vi "testSumin2.vi"() -> ()   [LabVIEW 2011]
panel:
  out "Image":T1(plugin-control)
  in  "DR/R parameter":T2
  out "BlkFilePath":path
  out "stim":i32
  out "Stimuli":i32
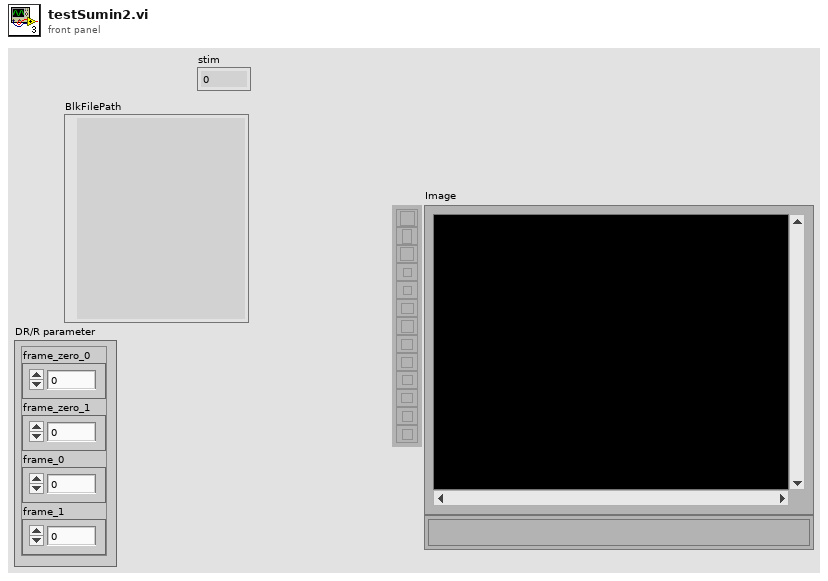
[diagram p1: front panel]
types:
  T1 = typedef "IMAQ Image.ctl" = refnum<image>
  T2 = cluster{"frame_zero_0":i32, "frame_zero_1":i32, "frame_0":i32, "frame_1":i32}
  T3 = typedef "Image Type" = u32
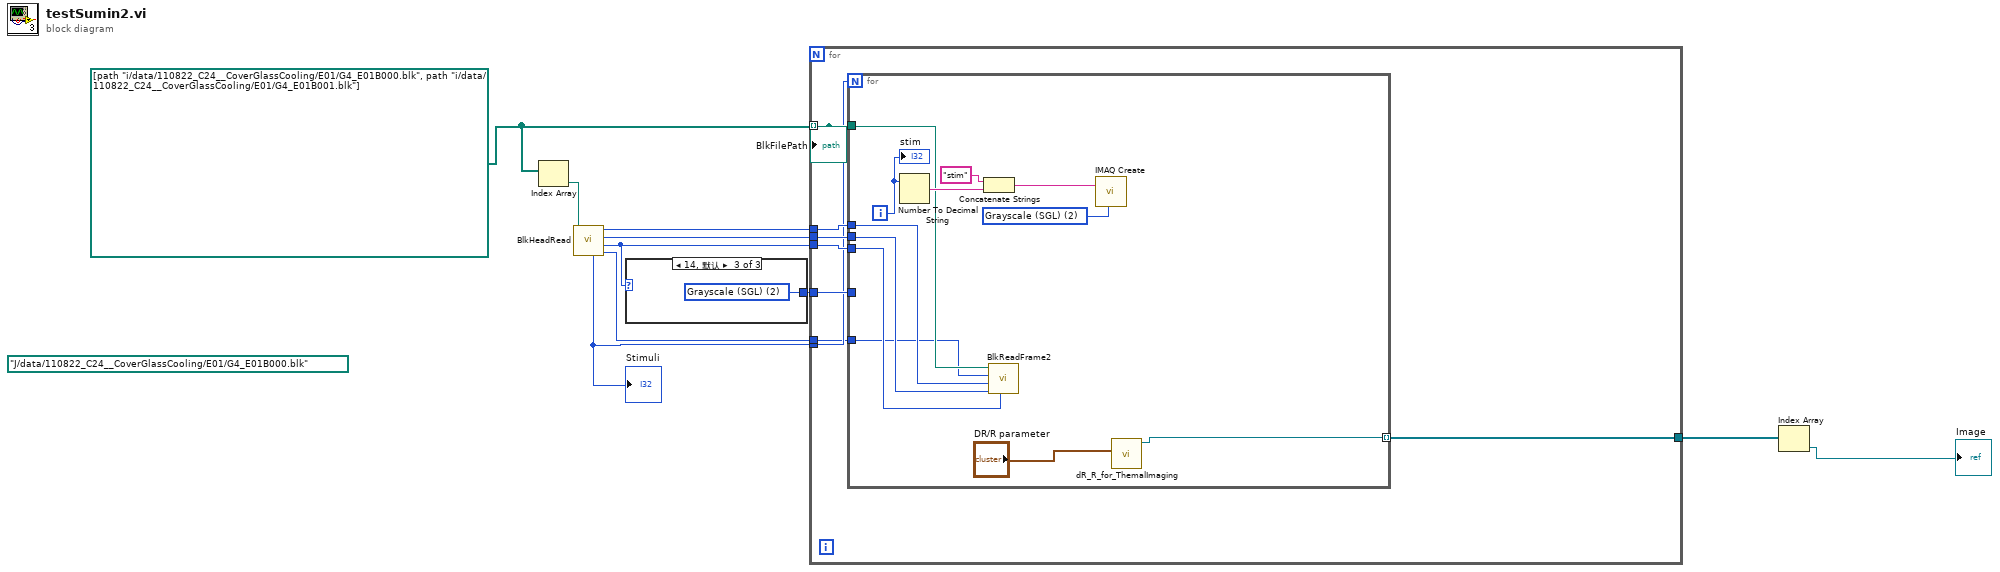
[diagram p0: block diagram]
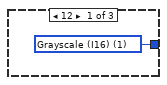
[diagram p2: hidden frame]
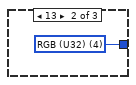
[diagram p3: hidden frame]
diagram:
  (unwired) path "J:/data/110822_C24__CoverGlassCooling/E01/G4_E01B000.blk" ("BlkFilePath")
  w4 = path[] [path "i:/data/110822_C24__CoverGlassCooling/E01/G4_E01B000.blk", path "i:/data/110822_C24__CoverGlassCooling/E01/G4_E01B001.blk"]
  n1 = Index Array(array=w4) -> (element=w3:path)  [unwired: 1 in]
  n2 = call "BlkHeadRead.vi"("BlkFilePath"=w3) -> ("FramesPerStim"=w7:i32, "datatype"=w8:i32, "FrameHeight"=w9:i32, "FrameWidth"=w10:i32, "Stimuli"=w6:i32)  [unwired: 6 in]
  "Stimuli" <- w6
  n3 = case shown="14, 默认" w8 {
    tunnel: [w11 w12 w13] -> w5
    frame 12 {
      w11 = T3 1 items=["Grayscale (U8)", "Grayscale (I16)", "Grayscale (SGL)", "Complex (CSG)", "RGB (U32)", "HSL (U32)", "RGB (U64)", "Grayscale (U16)"] ("Image Type")
    }
    frame 13 {
      w12 = T3 4 items=["Grayscale (U8)", "Grayscale (I16)", "Grayscale (SGL)", "Complex (CSG)", "RGB (U32)", "HSL (U32)", "RGB (U64)", "Grayscale (U16)"] ("Image Type")
    }
    frame 14, Default {
      w13 = T3 2 items=["Grayscale (U8)", "Grayscale (I16)", "Grayscale (SGL)", "Complex (CSG)", "RGB (U32)", "HSL (U32)", "RGB (U64)", "Grayscale (U16)"] ("Image Type")
    }
  }
  n4 = for {
    tunnel: w10 -> [w21]
    tunnel: w9 -> [w20]
    tunnel: w8 -> [w19]
    tunnel: w4 -> [w18] mode=indexing
    tunnel: w5 -> [w17]
    tunnel: w6 -> [w16]
    tunnel: w7 -> [w15]
    tunnel: [w14] -> w2
    n5 = for {
      N: w16 -> [_]
      tunnel: w18 -> [w30]
      tunnel: w21 -> [w29]
      tunnel: w20 -> [w28]
      tunnel: w19 -> [w27]
      tunnel: w17 -> [_]
      tunnel: w15 -> [w26]
      tunnel: [w22] -> w14 mode=indexing
      i -> [w33]
      w24 = T3 2 items=["Grayscale (U8)", "Grayscale (I16)", "Grayscale (SGL)", "Complex (CSG)", "RGB (U32)", "HSL (U32)", "RGB (U64)", "Grayscale (U16)"] ("Image Type")
      n6 = Number To Decimal String(number=w33) -> (decimal integer string=w32:string)  [unwired: 1 in]
      n7 = Concatenate Strings("stim" ("字符串"), w32) -> (w25:string)
      n8 = call "BlkReadFrame2.vi"("datatype"=w27, "FrameHeight"=w28, "FrameWidth"=w29, "frameNO."=w26, "BlkFilePath"=w30) -> ()  [unwired: 2 in, 3 out]
      n9 = call "IMAQ Create"("Image Name"=w25, "Image Type"=w24) -> ()  [unwired: 3 in, 2 out]
      n10 = call "dR_R_for_ThemalImaging.vi"("DR/R parameter"="DR/R parameter") -> ("Image Dst Out"=w22:T1)  [unwired: 10 in]
      "stim" <- w33
    }
    "BlkFilePath" <- w18
  }
  n11 = Index Array(array=w2) -> (element=→"Image":T1)  [unwired: 1 in]
